vi "Build Grid.vi"(11 "string Grid":string) -> (3 "unsigned byte array":u8[][](array[numeric]))   [LabVIEW 2023]
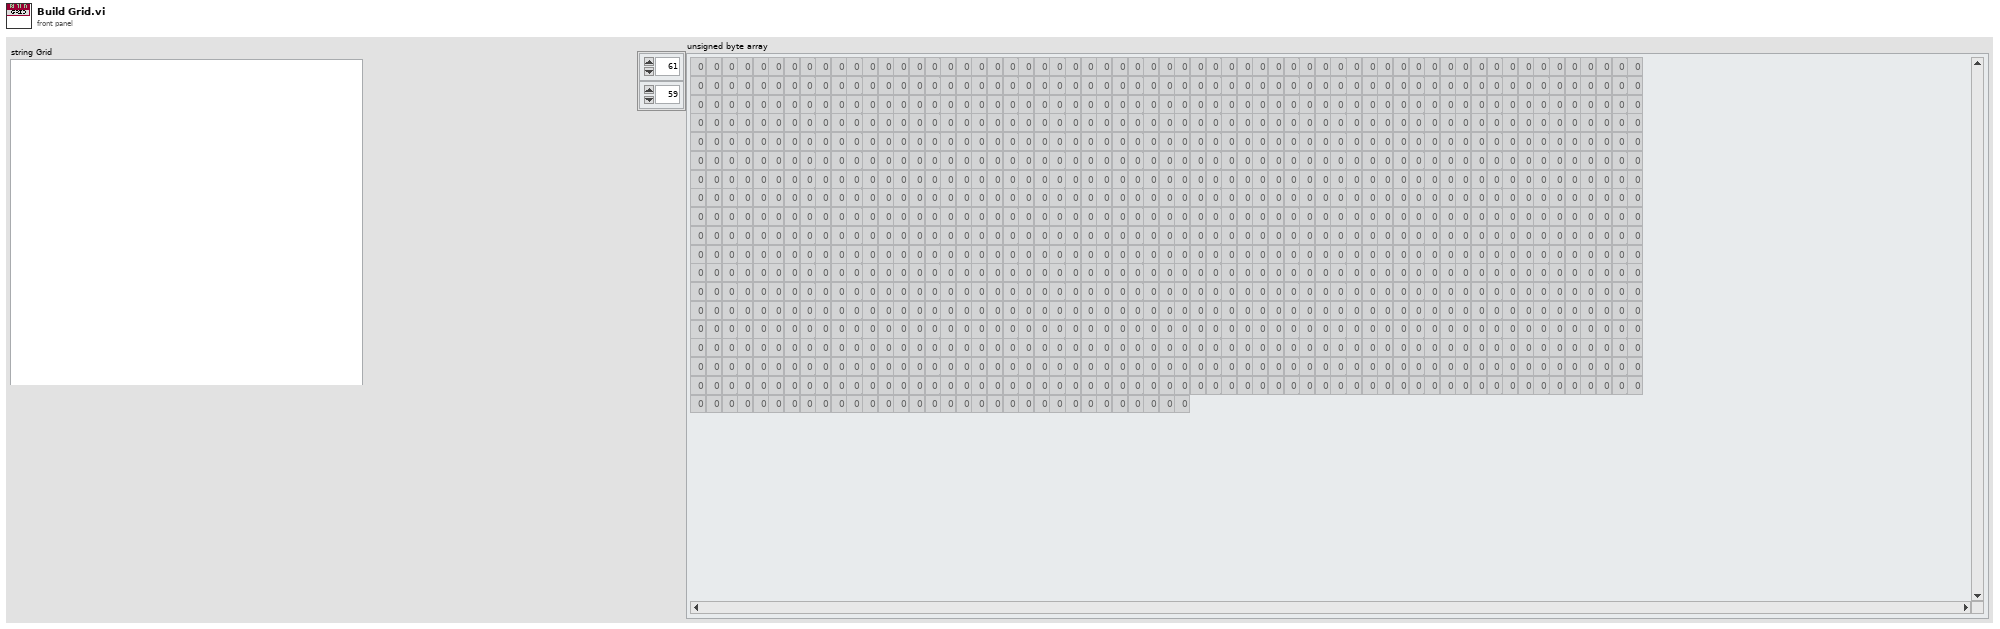
[diagram p1: front panel]
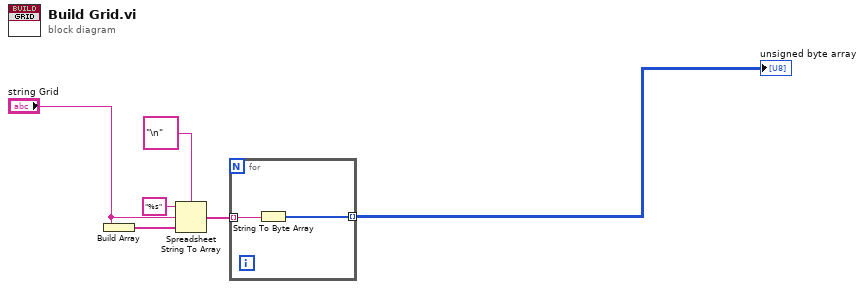
[diagram p0: block diagram]
diagram:
  n1 = Build Array("string Grid") -> (w2:string[])
  n2 = Spreadsheet String To Array(delimiter (Tab)="\n", format string="%s", spreadsheet string="string Grid", array type (2D Dbl)=w2) -> (array=w5:string[])
  n3 = for {
    tunnel: w5 -> [w8] mode=indexing
    tunnel: [w7] -> w1 mode=indexing
    n4 = String To Byte Array(string=w8) -> (unsigned byte array=w7:u8[])
  }
  "unsigned byte array" <- w1
